vi "OAT Demodulate Multiple Orders (Single Channel).vi"(0 "Y":dbl[](array[numeric]) format="%.2f", 1 "decimation factor":i32, 2 "reset? (True)":bool=TRUE, 3 "zero delay? (F)":bool, 5 "samples/rev":dbl=2.0 format="%.2f", 7 "samples/rev wanted":dbl=2.0 format="%.2f", 9 "orders (1.0)":dbl[](array[numeric])=[1.0] format="%.2f", 11 "time stamps in":dbl[](array[numeric]) format="%.2f", 12 "phase setting":T3, 13 "order info":T1 {"stop band attenuation" items=["72 dB", "96 dB", "120 dB"]; "bandwidth [order]" format="%.2f"}) -> (4 "magnitudes (RMS)":dbl[][](array[numeric]) format="%.2f", 6 "phase lag":dbl[][](array[numeric]) format="%.2f", 10 "samples/rev":dbl format="%.2f", 14 "speed profile":T2 {"speed [RPM]" format="%.2f"; "time [s]" format="%.2f"}, 15 "error out":errorcluster)   [LabVIEW 2017, in "SoundVib_Resampling.lvlib"]
uses:
  <vilib>/addons/Sound and Vibration/Order Analysis/Resample Order Tracking/SoundVib_Resampling.lvlib
  <vilib>/addons/Sound and Vibration/Order Analysis/Tach Process/SubVIs/speed profile.ctl
  <vilib>/addons/Sound and Vibration/Order Analysis/Tach Process/SoundVib_TachProcess.lvlib
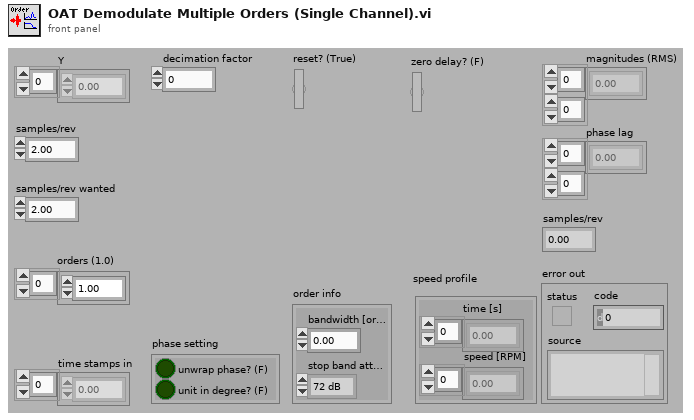
[diagram p1: front panel]
types:
  T1 = cluster{"bandwidth [order]":dbl, "stop band attenuation":u16}
  T2 = typedef "SoundVib_TachProcess.lvlib/speed profile.ctl" = cluster{"time [s]":dbl[], "speed [RPM]":dbl[]}
  T3 = cluster{"unwrap phase? (F)":bool, "unit in degree? (F)":bool}
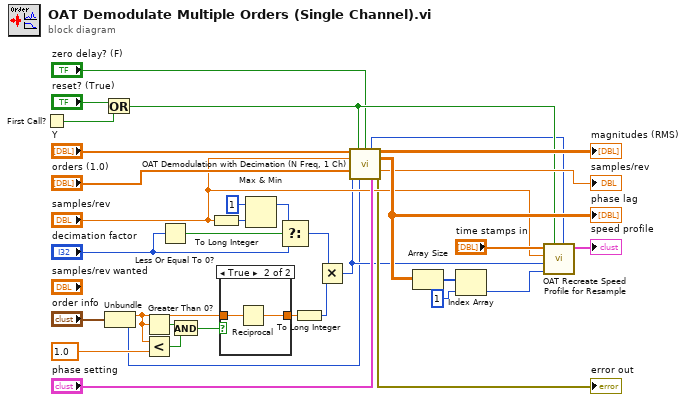
[diagram p0: block diagram]
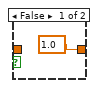
[diagram p2: hidden frame]
diagram:
  n1 = First Call?() -> (First Call?: T/F=w7:bool)
  n2 = Or(x="reset? (True)", y=w7) -> (x .or. y?=w6:bool)
  n3 = Unbundle("order info") -> ("bandwidth [order]"=w4:dbl, "stop band attenuation"=w3:u16)
  n4 = Greater Than 0?(x=w4) -> (x > 0?=w15:bool)
  n5 = Less?(x=w4, y=1.0) -> (x < y?=w14:bool)
  n6 = Less Or Equal To 0?(x="decimation factor") -> (x <= 0?=w32:bool)
  n7 = And(x=w15, y=w14) -> (x .and. y?=w13:bool)
  n8 = To Long Integer(number="samples/rev") -> (32bit integer=w28:i32)
  n9 = case shown="True" w13 {
    tunnel: w4 -> [_ w37]
    tunnel: [1.0 w36] -> w12
    frame False {
    }
    frame True {
      n10 = Reciprocal(x=w37) -> (1/x=w36:dbl)
    }
  }
  n11 = Max & Min(x=1, y=w28) -> (max(x,y)=w22:i32)  [unwired: 1 out]
  n12 = Select(t=w22, s=w32, f="decimation factor") -> (s? t:f=w10:i32)
  n13 = To Long Integer(number=w12) -> (32bit integer=w11:i32)
  n14 = Multiply(x=w10, y=w11) -> (x*y=w9:i32)
  n15 = call <vilib>:"OAT Demodulation with Decimation (N Freq, 1 Ch).vi"("x[n]"="Y", "reset? (True)"=w6, "zero delay? (F)"="zero delay? (F)", "fs"="samples/rev", "fc [Hz]"="orders (1.0)", "decimation factor"=w9, "stop band attenuation"=w3, "phase setting"="phase setting") -> ("lags"=w2:i32, "magnitudes (RMS)"=→"magnitudes (RMS)":dbl[][], "phase lag"=w26:dbl[][], "new fs [Hz]"=→"samples/rev":dbl, "error out"=→"error out":errorcluster)  [unwired: 3 in]
  "phase lag" <- w26
  n16 = Array Size(array=w26) -> (size(s)=w25:i32[])
  n17 = Index Array(array=w25, index=1) -> (element=w20:i32)
  n18 = call <vilib>:"OAT Recreate Speed Profile for Resample.vi"("lags"=w2, "init/continue (init:T)"=w6, "output length"=w20, "decimation factor"=w9, "sample / rev"="samples/rev", "time stamps in"="time stamps in") -> ("speed profile"=→"speed profile":T2)  [unwired: 5 in]
